vi "LM 3D Gaussian + Blinking ACF and gradient.vi"(3 "output control":T1, 4 "data":variant, 5 "X":dbl[](array[numeric]), 6 "a":dbl[](array[numeric])) -> (0 "error out":errorcluster, 1 "f'(X,a)":dbl[][](array[numeric]), 2 "f(X,a)":dbl[](array[numeric]))   [LabVIEW 2021, in "Fits.lvlib"]
doc: "This template is the starting point for creating a model function to be passed to the Nonlinear Curve Fit.vi."
uses:
  <vilib>/gmath/NumericalOptimization/LM_output select.ctl
  Fits.lvlib
  <vilib>/gmath/NI_Gmath.lvlib
panel:
  # "Parameters:\n\namplitude: A\ndiffusion time: t1\naspect ratio: w\nblinking fraction: b\nblinking time constant: t2"
  # "f(x) = 1 + A/(1+x/t1)/sqrt(1+x/t1/w^2)*(1- b + b*Exp(-x/t2)"
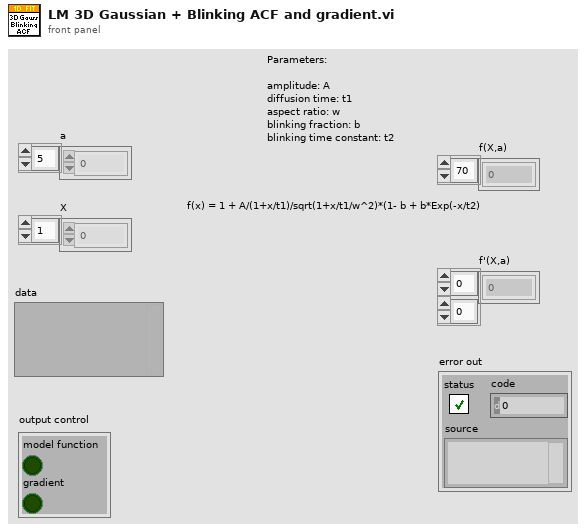
[diagram p1: front panel]
types:
  T1 = typedef "NI_Gmath.lvlib/LM_output select.ctl" = cluster{"model function":bool, "gradient":bool}
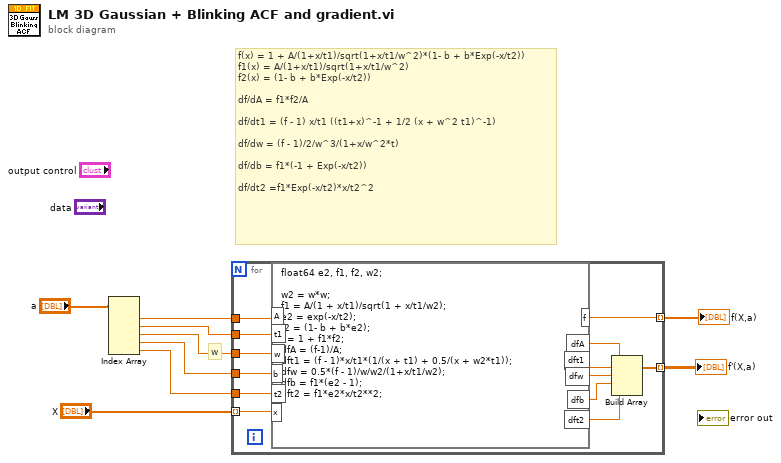
[diagram p0: block diagram]
diagram:
  # "w"
  # "f(x) = 1 + A/(1+x/t1)/sqrt(1+x/t1/w^2)*(1- b + b*Exp(-x/t2))\nf1(x) = A/(1+x/t1)/sqrt(1+x/t1/w^2)\nf2(x) = (1- b + b*Exp(-x/t2))\n\ndf/dA = f1*f2/A\n\ndf/dt1 = (f - 1) x/t1 ((t1+x)^-1 + 1/2 (x + w^2 t1)^-1)\n\ndf/dw = (f - 1)/2/w^3/(1+x/w^2*t)\n\ndf/db = f1*(-1 + Exp(-x/t2))\n\ndf/dt2 =f1*Exp(-x/t2)*x/t2^2"
  n1 = Index Array(array="a") -> (element #1=w5:dbl, element #2=w4:dbl, element #3=w1:dbl, element #4=w2:dbl, element #5=w3:dbl)  [unwired: 5 in]
  n2 = for {
    tunnel: w5 -> [w21]
    tunnel: w4 -> [w22]
    tunnel: "X" -> [w20] mode=indexing
    tunnel: [w19] -> w7 mode=indexing
    tunnel: [w16] -> w6 mode=indexing
    tunnel: w2 -> [w15]
    tunnel: w3 -> [w14]
    tunnel: w1 -> [w11]
    n3 = formula code="float64 e2, f1, f2, w2;\n\nw2 = w*w;\nf1 = A/(1 + x/t1)/sqrt(1 + x/t1/w2);\ne2 = exp(-x/t2);\nf2 = (1- b + b*e2);\nf = 1 + f1*f2;\ndfA = (f-1)/A;\ndft1 = (f - 1)*x/t1*(1/(x + t1) + 0.5/(x + w2*t1));\ndfw = 0.5*(f - 1)/w/w2/(1+x/t1/w2);\ndfb = f1*(e2 - 1);\ndft2 = f1*e2*x/t2**2;"("A"=w21, "t1"=w22, "x"=w20, "b"=w15, "t2"=w14, "w"=w11) -> ("f"=w19:dbl, "dfA"=w18:dbl, "dft1"=w17:dbl, "dfb"=w13:dbl, "dft2"=w12:dbl, "dfw"=w10:dbl)
    n4 = Build Array(w18, w17, w10, w13, w12) -> (w16:dbl[])
  }
  "f(X,a)" <- w7
  "f'(X,a)" <- w6
